vi "Error Logger.vi"(7 "Action":T1(ring), 8 "error in":errorcluster, 9 "Buffer(lines)":i32=5000, 10 "Log File":path) -> (0 "error out":errorcluster, 3 "Log":string)   [LabVIEW 2020]
uses:
  Main Globals.vi
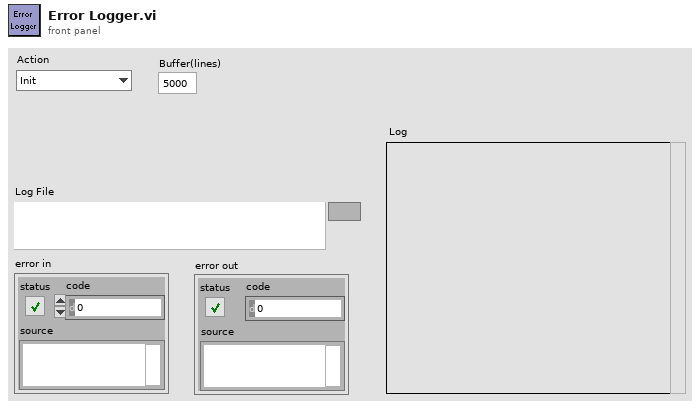
[diagram p1: front panel]
types:
  T1 = enum16{"Init", "Reset", "Read", "Update", "Close"}
  T2 = enum16{"open", "replace", "create", "open or create", "replace or create", "replace or create with confirmation"}
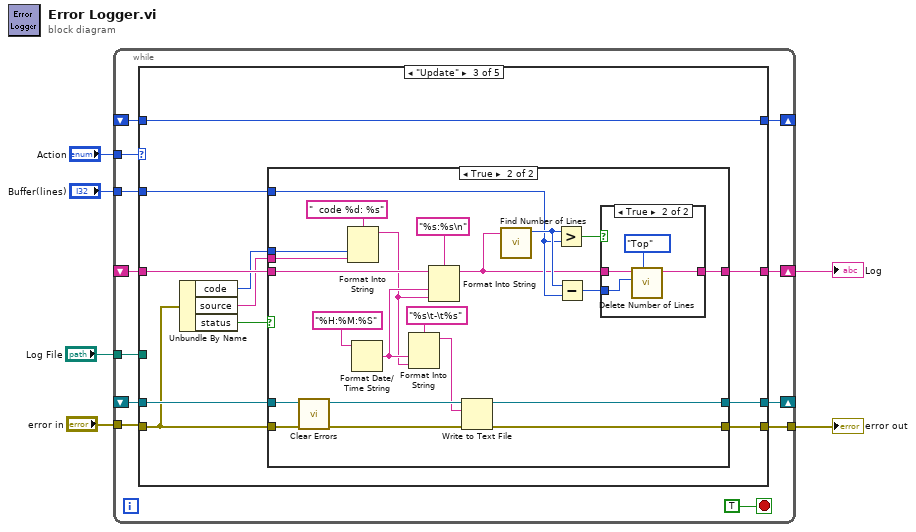
[diagram p0: block diagram]
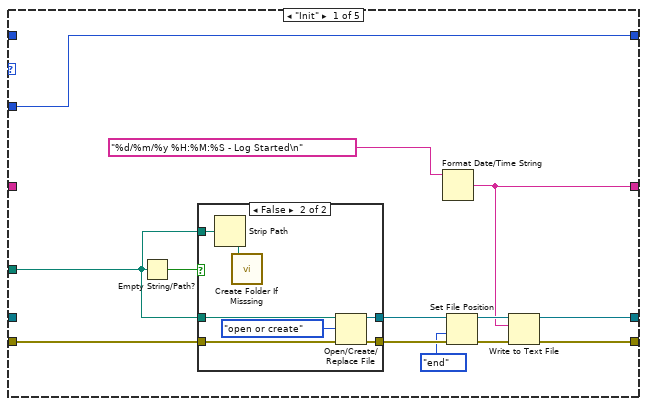
[diagram p2: hidden frame]
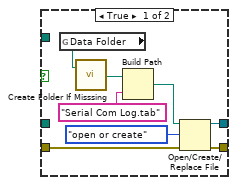
[diagram p3: hidden frame]
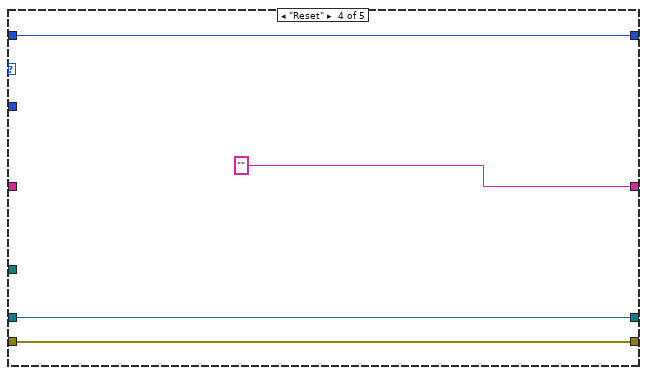
[diagram p7: hidden frame]
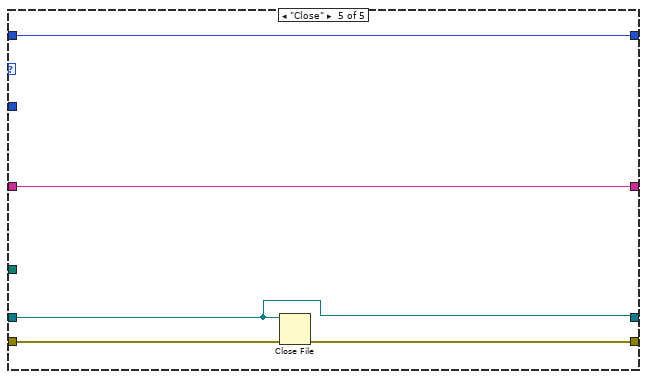
[diagram p8: hidden frame]
diagram:
  n1 = while {
    tunnel: "error in" -> [w17]
    tunnel: [w14] -> w5
    tunnel: "Action" -> [w16]
    tunnel: "Log File" -> [w15]
    shift-right: [w13] -> _
    shift-left: _ -> [w12]
    shift-right: [w11] -> w1
    shift-left: _ -> [w10]
    tunnel: "Buffer(lines)" -> [w9]
    shift-right: [w8] -> _
    shift-left: _ -> [w7]
    stop <- TRUE stop-if-true
    n2 = case shown="\"Update\"" w16 {
      tunnel: w17 -> [w30 w49 w54 w92 w98]
      tunnel: w15 -> [w29 _ _ _ _]
      tunnel: [w23 w49 w56 w92 w97] -> w14
      tunnel: [w22 w48 w57 w93 w96] -> w13
      tunnel: w12 -> [_ w48 w61 w93 w96]
      tunnel: [w20 w50 w58 "" ("Resulting String") w99] -> w11
      tunnel: w10 -> [_ w50 w60 _ w99]
      tunnel: w9 -> [w19 _ w59 _ _]
      tunnel: [w19 w47 w55 w91 w95] -> w8
      tunnel: w7 -> [_ w47 w55 w91 w95]
      frame "Init" {
        n3 = Empty String/Path?(string/path=w29) -> (empty?=w31:bool)
        n4 = case shown="False" w31 {
          tunnel: w30 -> [w34 w45]
          tunnel: [w33 w44] -> w28
          tunnel: w29 -> [_ w42]
          tunnel: w29 -> [_ w41]
          tunnel: [w32 w40] -> w27
          frame True {
            n5 = global read "Main Globals.vi" "Data Folder"() -> (w39:path)
            n6 = call "Create Folder If Misssing.vi"("Path In"=w39) -> ("Path Out"=w38:path)  [unwired: 1 in, 1 out]
            n7 = Build Path(base path=w38, name or relative path="Serial Com Log.tab") -> (appended path=w36:path)
            n8 = Open/Create/Replace File(file path (use dialog)=w36, error in=w34, operation (0:open)=T2."open or create") -> (refnum out=w32:refnum<file>, error out=w33:errorcluster)  [unwired: 3 in, 1 out]
          }
          frame False {
            n9 = Strip Path(path=w42) -> (stripped path=w43:path)  [unwired: 1 out]
            n10 = call "Create Folder If Misssing.vi"("Path In"=w43) -> ()  [unwired: 1 in, 2 out]
            n11 = Open/Create/Replace File(file path (use dialog)=w41, error in=w45, operation (0:open)=T2."open or create") -> (refnum out=w40:refnum<file>, error out=w44:errorcluster)  [unwired: 3 in, 1 out]
          }
        }
        n12 = Format Date/Time String(time format string (%c)="%d/%m/%y %H:%M:%S - Log Started\n") -> (date/time string=w20:string)  [unwired: 2 in]
        n13 = Set File Position(refnum=w27, from (0:start)=enum16{"start", "end", "current"}."end", error in=w28) -> (refnum out=w25:refnum<file>, error out=w21:errorcluster)  [unwired: 1 in]
        n14 = Write to Text File(file (use dialog)=w25, text=w20, error in=w21) -> (refnum out=w22:refnum<file>, error out=w23:errorcluster)  [unwired: 1 in, 1 out]
      }
      frame "Read" {
      }
      frame "Update" {
        n15 = Unbundle By Name(w54) -> ("code"=w53:i32, "source"=w52:string, "status"=w51:bool)
        n16 = case shown="True" w51 {
          tunnel: w61 -> [w63 w83]
          tunnel: w60 -> [w62 w81]
          tunnel: w59 -> [_ w78]
          tunnel: [w62 w75] -> w58
          tunnel: [w63 w73] -> w57
          tunnel: [w64 w72] -> w56
          tunnel: w54 -> [w64 w70]
          tunnel: w53 -> [_ w66]
          tunnel: w52 -> [_ w65]
          frame False {
            # "no error"
          }
          frame True {
            n17 = call <vilib>:"Clear Errors.vi"("error in (no error)"=w70) -> ("error out"=w67:errorcluster)  [unwired: 5 in, 1 out]
            n18 = Format Into String(format string="  code %d: %s", w66, w65) -> (resulting string=w68:string)  [unwired: 2 in, 1 out]
            n19 = Format Date/Time String(time format string (%c)="%H:%M:%S") -> (date/time string=w71:string)  [unwired: 2 in]
            n20 = Format Into String(format string="%s\t-\t%s", w71, w68) -> (resulting string=w82:string)  [unwired: 2 in, 1 out]
            n21 = Format Into String(format string="%s:%s\n", initial string=w81, w71, w68) -> (resulting string=w76:string)  [unwired: 1 in, 1 out]
            n22 = Write to Text File(file (use dialog)=w83, text=w82, error in=w67) -> (refnum out=w73:refnum<file>, error out=w72:errorcluster)  [unwired: 1 in, 1 out]
            n23 = call "Find Number of Lines.vi"("String"=w76) -> ("Number of Lines"=w79:i32)  [unwired: 10 in]
            n24 = Greater?(x=w79, y=w78) -> (0:w80:bool)
            n25 = Subtract(x=w79, y=w78) -> (x-y=w77:i32)
            n26 = case shown="True" w80 {
              tunnel: w77 -> [_ w89]
              tunnel: w76 -> [w86 w90]
              tunnel: [w86 w88] -> w75
              frame False {
              }
              frame True {
                n27 = call "Delete Number of Lines.vi"("Position"=enum16{"Top", "Bottom", "Line N"}."Top", "Number of Lines"=w89, "String"=w90) -> ("Resulting String"=w88:string)  [unwired: 8 in]
              }
            }
          }
        }
      }
      frame "Reset" {
      }
      frame "Close" {
        n28 = Close File(refnum=w96, error in=w98) -> (error out=w97:errorcluster)  [unwired: 1 out]
      }
    }
  }
  "error out" <- w5
  "Log" <- w1
